vi "Мажор +.vi"() -> ()   [LabVIEW 2017]
panel:
  out "Декодированное сообщение 3":dbl[](array[numeric])
  out "sum 4":i16
  out "sum 3":i16
  out "s? t:f":dbl
  out "element":dbl
  out "После ошибки":dbl[](array[numeric])
  out "2-х массив на выходе 3":dbl[][](array[numeric])
  out "см. 1.5":dbl[][](array[numeric])
  out "До ошибки":dbl[](array[numeric])
  in  "Кол-во копий":i32=5
  out "Массиве":dbl[](array[numeric])
  in  "Кол-во элементов":i32=16
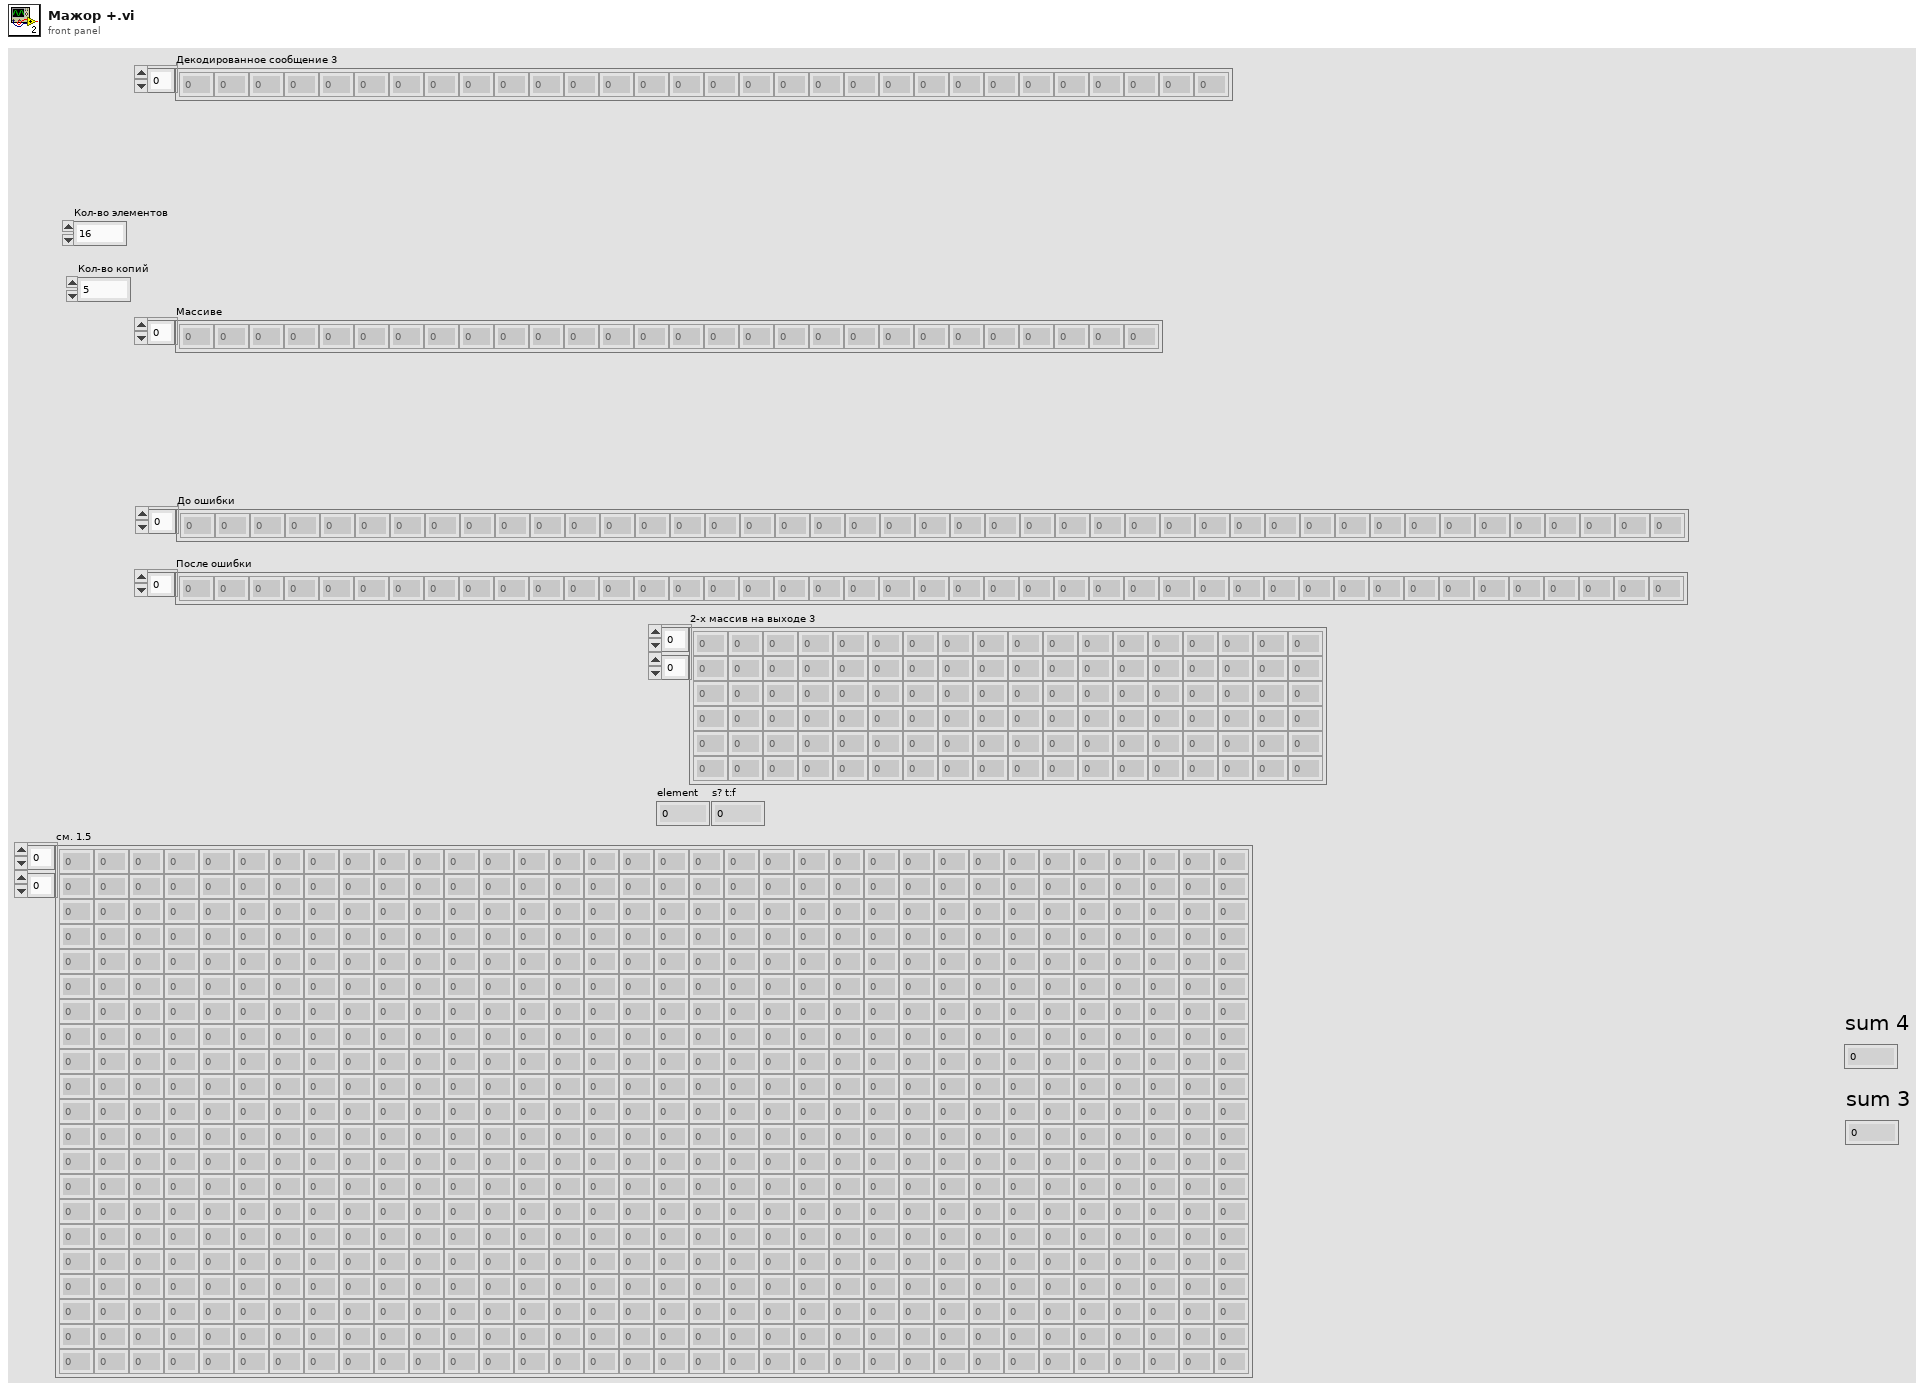
[diagram p1: front panel]
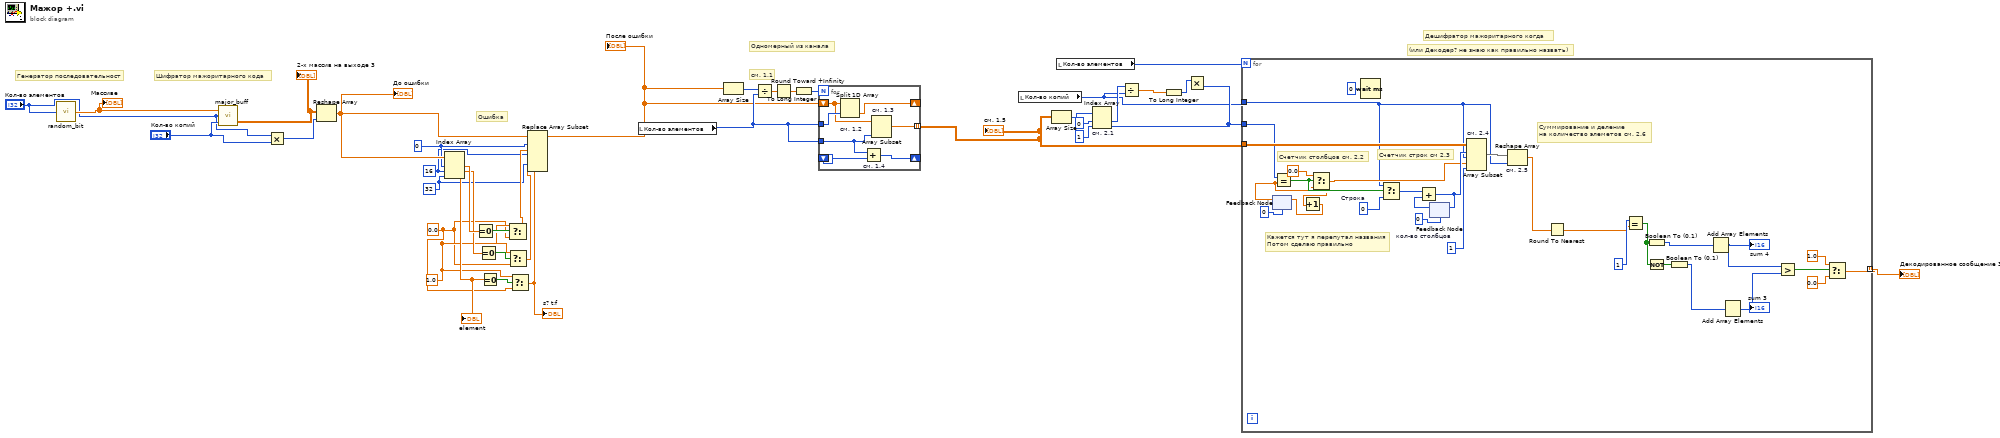
[diagram p0: block diagram]
diagram:
  w9 = 1.0
  w8 = 0.0
  w2 = 32
  w3 = 16
  w4 = 0
  # "Ошибка"
  # "Одномерный из канала"
  # "см. 1.1"
  # "(или Декодер? не знаю как правильно назвать)"
  # "Дешифратор мажоритарного когда"
  # "Шифратор мажоритарного кода"
  # "Генератор последовательност"
  n1 = call "random_bit.vi"("Количество бит"="Кол-во элементов") -> ("Биты на выходе 1"=w37:dbl[])
  "Массиве" <- w37
  n2 = call "major_buff.vi"("Кол-во копий"="Кол-во копий", "Размер окна"="Кол-во элементов", "Биты на выходе 1"=w37) -> ("Подготовленный к отправке мажоритарный код"=w18:dbl[][])  [unwired: 1 out]
  "2-х массив на выходе 3" <- w18
  n3 = Multiply(x="Кол-во элементов", y="Кол-во копий") -> (x*y=w36:i32)
  n4 = Reshape Array(w18, w36) -> (w16:dbl[])
  "До ошибки" <- w16
  n5 = Index Array(array=w16, index #1=w4, index #2=w3, index #3=w2) -> (element #1=w15:dbl, element #2=w14:dbl, element #3=w13:dbl)
  "element" <- w13
  n6 = Equal To 0?(x=w15) -> (x = 0?=w12:bool)
  n7 = Equal To 0?(x=w14) -> (x = 0?=w11:bool)
  n8 = Equal To 0?(x=w13) -> (x = 0?=w10:bool)
  n9 = Select(t=w9, s=w12, f=w8) -> (s? t:f=w7:dbl)
  n10 = Select(t=w9, s=w11, f=w8) -> (s? t:f=w6:dbl)
  n11 = Select(t=w9, s=w10, f=w8) -> (s? t:f=w5:dbl)
  "s? t:f" <- w5
  n12 = Replace Array Subset(array=w16, new element #1=w7, index #1=w4, new element #2=w6, index #2=w3, new element #3=w5, index #3=w2) -> (w21:dbl[])
  "После ошибки" <- w21
  n13 = local read "Кол-во элементов"() -> (w27:i32)
  n14 = Array Size(array=w21) -> (size(s)=w26:i32)
  n15 = Divide(x=w26, y=w27) -> (x/y=w25:dbl)
  n16 = Round Toward +Infinity(x=w25) -> (ceil(x): smallest int >= x=w24:dbl)
  n17 = To Long Integer(number=w24) -> (32bit integer=w23:i32)
  n18 = for {
    N: w23 -> [_]
    shift-right: [w44] -> _
    shift-left: w21 -> [w42]
    tunnel: w27 -> [w43]
    shift-right: [w40] -> _
    shift-left: _ -> [w39]
    tunnel: w27 -> [w41]
    tunnel: [w38] -> w17 mode=indexing
    n19 = Split 1D Array "см. 1.2"(array=w42, index=w43) -> (second subarray=w44:dbl[])  [unwired: 1 out]
    n20 = Add "см. 1.4"(x=w41, y=w39) -> (x+y=w40:i32)
    n21 = Array Subset "см. 1.3"(array=w42, length=w41) -> (w38:dbl[])  [unwired: 1 in]
  }
  "см. 1.5" <- w17
  n22 = local read "Кол-во копий"() -> (w28:i32)
  n23 = Array Size(array=w17) -> (size(s)=w35:i32[])
  n24 = local read "Кол-во элементов"() -> (w22:i32)
  n25 = Index Array "см. 2.1"(array=w35, index #1=0 ("index"), index #2=1 ("index")) -> (element #1=w32:i32, element #2=w31:i32)
  n26 = Divide(x=w32, y=w28) -> (x/y=w30:dbl)
  n27 = To Long Integer(number=w30) -> (32bit integer=w29:i32)
  n28 = Multiply(x=w29, y=w31) -> ()  [unwired: 1 out]
  n29 = for {
    N: w22 -> [_]
    tunnel: w17 -> [w73]
    tunnel: w31 -> [w65]
    tunnel: w28 -> [w58]
    tunnel: [w48] -> w1 mode=indexing
    w72 = 1  # кол-во столбцов
    w63 = 0  # Строка
    # "Суммирование и деление \nна количество элеметов см. 2.6"
    # "Кажется тут я перепутал названия  \nПотом сделаю правильно"
    # "Счетчик строк см 2.3"
    # "Счетчик столбцов см. 2.2"
    n30 = feedback #1(0) -> (w61:dbl)
    n31 = Equal?(x=w65, y=w61) -> (x = y?=w67:bool)
    n32 = Select(t=0.0, s=w67, f=w61) -> (s? t:f=w60:dbl)
    n33 = Increment(x=w60) -> (x+1=w59:dbl)
    n34 = feedback-in #1(w59) -> ()
    n35 = Wait (ms)(milliseconds to wait=u32 0) -> ()  [unwired: 1 out]
    n36 = Select(t=w58, s=w67, f=w63) -> (s? t:f=w64:i32)
    n37 = feedback #2(0) -> (w66:i32)
    n38 = Add(x=w64, y=w66) -> (x+y=w62:i32)
    n39 = feedback-in #2(w62) -> ()
    n40 = Array Subset "см. 2.4"(array=w73, index (row)=w62, length (row)=w58, index (col)=w60, length (col)=w72) -> (w74:dbl[][])
    n41 = Reshape Array "см. 2.5"(w74, w58) -> (w45:dbl[])
    n42 = Round To Nearest(number=w45) -> (nearest integer value=w49:dbl[])
    n43 = Equal?(x=1, y=w49) -> (x = y?=w51:bool[])
    n44 = Boolean To (0,1)(Boolean=w51) -> (0, 1=w47:i16[])
    n45 = Not(x=w51) -> (.not. x?=w52:bool[])
    n46 = Boolean To (0,1)(Boolean=w52) -> (0, 1=w46:i16[])
    n47 = Add Array Elements(numeric array=w47) -> (sum=w54:i16)
    "sum 4" <- w54
    n48 = Add Array Elements(numeric array=w46) -> (sum=w53:i16)
    "sum 3" <- w53
    n49 = Greater?(x=w54, y=w53) -> (0:w57:bool)
    n50 = Select(t=1.0, s=w57, f=0.0) -> (s? t:f=w48:dbl)
  }
  "Декодированное сообщение 3" <- w1
